vi "Anritsu VNA Read IFBW.vi"(6 "Channel":i8=1 min=1 max=99 step=1, 7 "Anritsu VNA":T1, 8 "error in (no error)":errorcluster, 11 "VISA Resource Name":refnum<visa-resource-name>) -> (0 "error out":errorcluster, 2 "IFBW, Hz":dbl=3000.0, 3 "dup VISA Resource Name":refnum<visa-resource-name>)   [LabVIEW 2011]
doc: "This Vi for the HP8753B Network Analyzer is used to set averaging, smoothing, and the IF bandwidth."
uses:
  TypeDefs/Anritsu VNA Instrument Info.ctl
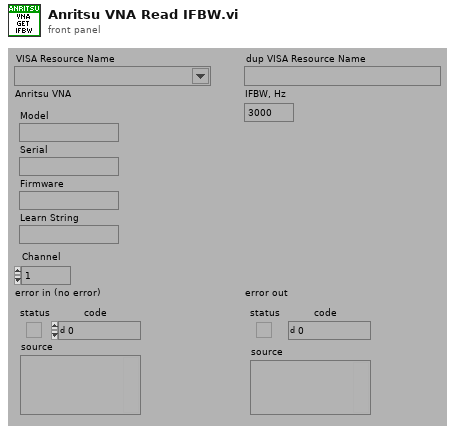
[diagram p1: front panel]
types:
  T1 = typedef "Anritsu VNA Instrument Info.ctl" = cluster{"Model":string, "Serial":string, "Firmware":string, "Learn String":string}
  T2 = typedef "Anritsu VNA Model.ctl" = enum16{"Not Supported", "37XXXX", "MS20XXX", "MS462XX", "MS464XX"}
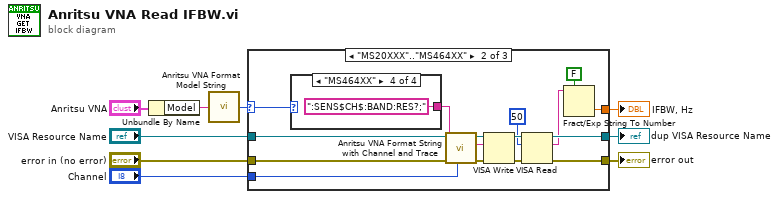
[diagram p0: block diagram]
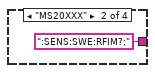
[diagram p4: hidden frame]
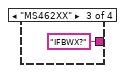
[diagram p5: hidden frame]
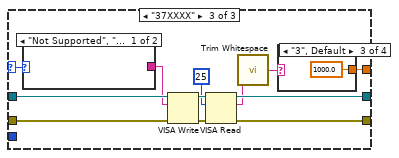
[diagram p6: hidden frame]
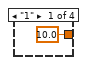
[diagram p7: hidden frame]
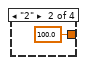
[diagram p8: hidden frame]
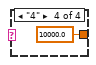
[diagram p9: hidden frame]
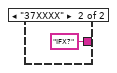
[diagram p10: hidden frame]
diagram:
  n1 = Unbundle By Name("Anritsu VNA") -> ("Model"=w3:string)
  n2 = call "Anritsu VNA Format Model String.vi"("Model"=w3) -> ("Model"=w2:T2)
  n3 = case shown="\"MS20XXX\"..\"MS464XX\"" w2 {
    selector: w2 -> [_ w15 w32]
    tunnel: "VISA Resource Name" -> [w11 w25 w40]
    tunnel: "error in (no error)" -> [w10 w24 w39]
    tunnel: [w11 w22 w37] -> w7
    tunnel: [w10 w18 w34] -> w6
    tunnel: [_ w16 w29] -> w5
    tunnel: "Channel" -> [_ w12 _]
    frame "Not Supported" {
    }
    frame "MS20XXX".."MS464XX" {
      n4 = case shown="\"MS464XX\"" w15 {
        tunnel: [_ ":SENS:SWE:RFIM?;" "IFBWX?" ":SENS$CH$:BAND:RES?;"] -> w13
        frame "Not Supported", "37XXXX" {
        }
        frame "MS20XXX" {
        }
        frame "MS462XX" {
        }
        frame "MS464XX" {
        }
      }
      n5 = call "Anritsu VNA Format String with Channel and Trace.vi"("Channel"=w12, "String"=w13) -> ("String Out"=w14:string)  [unwired: 1 in, 6 out]
      n6 = VISA Write(VISA resource name=w25, write buffer=w14, error in (no error)=w24) -> (VISA resource name out=w23:refnum<visa-resource-name>, error out=w19:errorcluster)  [unwired: 1 out]
      n7 = VISA Read(VISA resource name=w23, byte count=u32 50, error in (no error)=w19) -> (VISA resource name out=w22:refnum<visa-resource-name>, read buffer=w17:string, error out=w18:errorcluster)  [unwired: 1 out]
      n8 = Fract/Exp String To Number(use system decimal point (T)=FALSE, string=w17) -> (number=w16:dbl)  [unwired: 3 out]
    }
    frame "37XXXX" {
      n9 = case shown="\"Not Supported\", \"MS20XXX\"..\"MS464XX\"" w32 {
        tunnel: [_ "IFX?"] -> w33
        frame "Not Supported", "MS20XXX".."MS464XX" {
        }
        frame "37XXXX" {
        }
      }
      n10 = VISA Write(VISA resource name=w40, write buffer=w33, error in (no error)=w39) -> (VISA resource name out=w38:refnum<visa-resource-name>, error out=w35:errorcluster)  [unwired: 1 out]
      n11 = VISA Read(VISA resource name=w38, byte count=u32 25, error in (no error)=w35) -> (VISA resource name out=w37:refnum<visa-resource-name>, read buffer=w31:string, error out=w34:errorcluster)  [unwired: 1 out]
      n12 = call <vilib>:"Trim Whitespace.vi"("string"=w31) -> ("trimmed string"=w30:string)  [unwired: 1 in]
      n13 = case shown="\"3\", Default" w30 {
        tunnel: [10.0 ("number") 100.0 ("number") 1000.0 ("number") 10000.0 ("number")] -> w29
        frame "1" {
        }
        frame "2" {
        }
        frame "3", Default {
        }
        frame "4" {
        }
      }
    }
  }
  "error out" <- w6
  "dup VISA Resource Name" <- w7
  "IFBW, Hz" <- w5
